vi "get_config_cluster.vi"(8 "error in (no error)":errorcluster, 11 "SignalWriterMH110203USBStepperMotor in":refnum<class "SignalWriterMH110203USBStepperMotor.lvclass">) -> (0 "error out":errorcluster, 2 "config cluster (variant)":variant, 3 "SignalWriterMH110203USBStepperMotor out":refnum<class "SignalWriterMH110203USBStepperMotor.lvclass">)   [LabVIEW 2010, in "SignalWriterMH110203USBStepperMotor.lvclass"]
uses:
  SignalWriterMH110203USBStepperMotor.lvclass
  SignalWriterMH110203USBStepperMotor.lvclass/SignalWriterMH110203USBStepperMotor.ctl
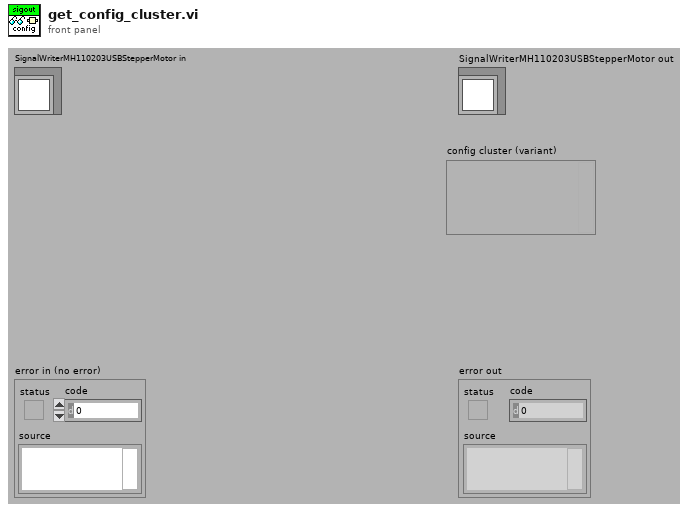
[diagram p1: front panel]
types:
  T1 = typedef "SignalWriterMH110203USBStepperMotor.lvclass/config_data_cluster.ctl" = cluster{"maximum output value":dbl, "minimum output value":dbl, "step":u8, "speed":dbl, "axis":i32}
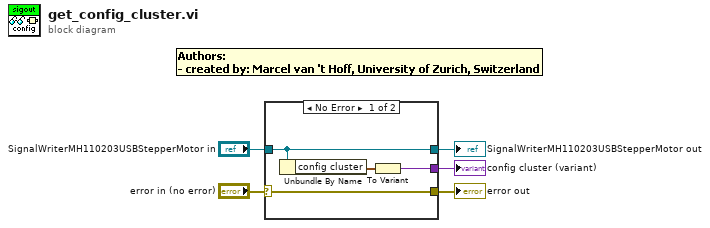
[diagram p0: block diagram]
diagram:
  n1 = case shown="No Error" "error in (no error)" {
    selector: "error in (no error)" -> [w9 w10]
    tunnel: "SignalWriterMH110203USBStepperMotor in" -> [w8 w11]
    tunnel: [w9 w10] -> w3
    tunnel: [w8 w11] -> w1
    tunnel: [w6 _] -> w2
    frame No Error {
      n2 = Unbundle By Name(w8) -> ("config cluster"=w7:T1)
      n3 = To Variant(anything=w7) -> (Variant=w6:variant)
    }
    frame Error {
    }
  }
  "error out" <- w3
  "SignalWriterMH110203USBStepperMotor out" <- w1
  "config cluster (variant)" <- w2
